vi "Fitness Core Override.vi"(8 "error in (no error)":errorcluster, 9 "Target Binary String (LSb[0] - MSb[n-1])":bool[](array[boolean]), 10 "Parent Binary String (LSb[0] - MSb[n-1])":bool[](array[boolean]), 11 "IChromosome in":refnum<class "IChromosome.lvclass">) -> (0 "error out":errorcluster, 2 "Fitness Score":dbl, 3 "IChromosome out":refnum<class "IChromosome.lvclass">)   [LabVIEW 2016, in "IChromosome.lvclass"]
uses:
  IChromosome.lvclass
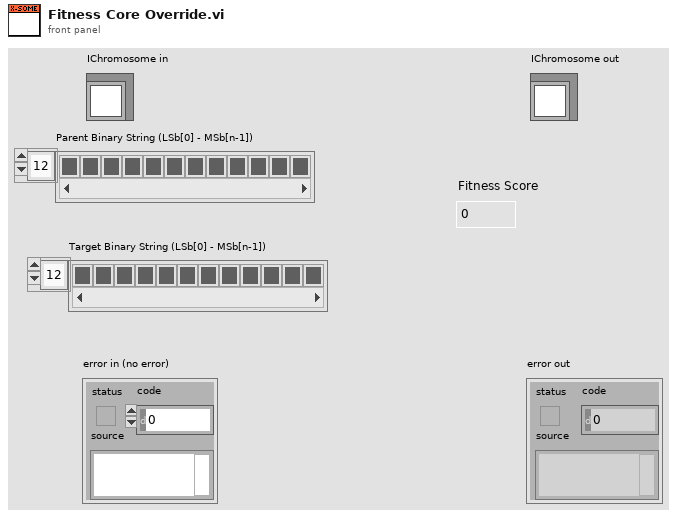
[diagram p1: front panel]
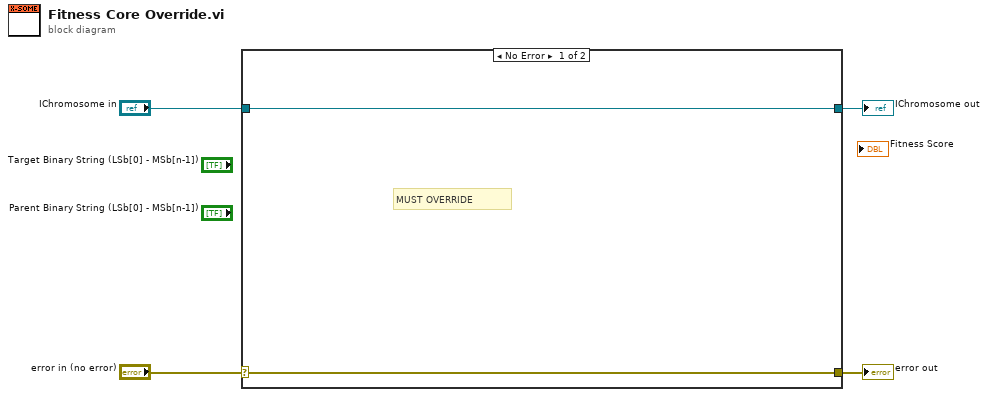
[diagram p0: block diagram]
diagram:
  n1 = case shown="No Error" "error in (no error)" {
    selector: "error in (no error)" -> [w5 w8]
    tunnel: [w5 w8] -> w3
    tunnel: [w6 w7] -> w1
    tunnel: "IChromosome in" -> [w6 w7]
    frame No Error {
      # "MUST OVERRIDE"
    }
    frame Error {
    }
  }
  "error out" <- w3
  "IChromosome out" <- w1
